vi "DRIVE_SIMPLE.vi"(10 "argv":string[](array[string]), 11 "args":u8) -> ()   [LabVIEW 2011]
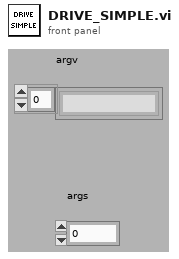
[diagram p1: front panel]
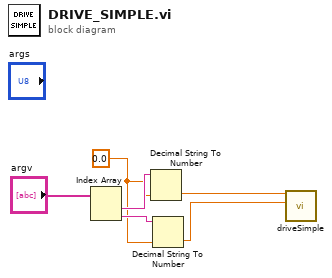
[diagram p0: block diagram]
diagram:
  w3 = 0.0
  n1 = Index Array(array="argv") -> (element #1=w5:string, element #2=w4:string)  [unwired: 2 in]
  n2 = Decimal String To Number(string=w5, default (0L)=w3) -> (number=w2:dbl)  [unwired: 1 in, 1 out]
  n3 = Decimal String To Number(string=w4, default (0L)=w3) -> (number=w1:dbl)  [unwired: 1 in, 1 out]
  n4 = call "driveSimple.vi"("Speed (ft/sec)"=w1, "Distance"=w2) -> ()  [unwired: 10 in]
